vi "Write UUID.vi"(8 "error in (no error)":errorcluster, 10 "UUID":string, 11 "UI View in":refnum<class "UI View.lvclass">) -> (0 "error out":errorcluster, 3 "UI View out":refnum<class "UI View.lvclass">)   [LabVIEW 2013, in "SET Project Editor.lvlib" / "UI View.lvclass"]
uses:
  UI View.lvclass
  UI View.lvclass/UI View.ctl
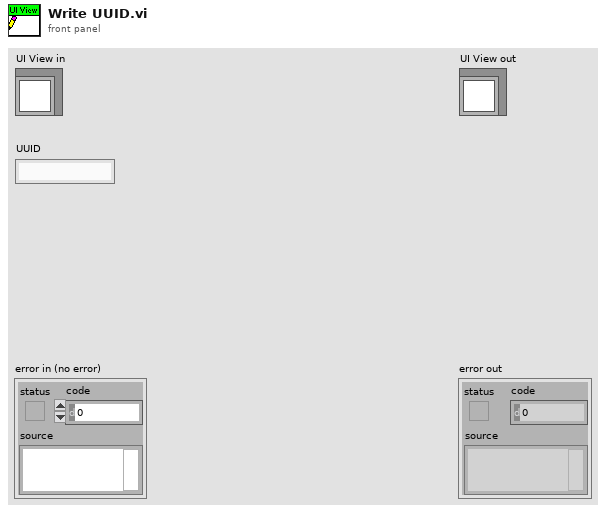
[diagram p1: front panel]
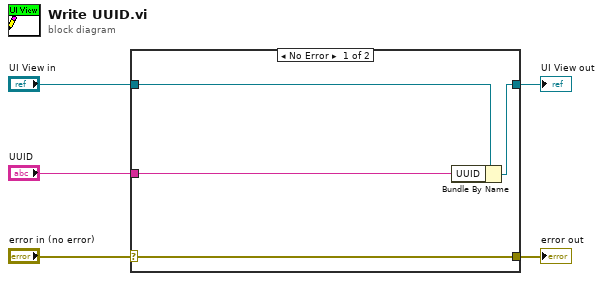
[diagram p0: block diagram]
diagram:
  n1 = case shown="No Error" "error in (no error)" {
    selector: "error in (no error)" -> [w9 w10]
    tunnel: [w9 w10] -> w4
    tunnel: [w7 w11] -> w2
    tunnel: "UI View in" -> [w8 w11]
    tunnel: "UUID" -> [w6 _]
    frame No Error {
      n2 = Bundle By Name(cluster=w8, "UUID"=w6) -> (w7:refnum<class "UI View.lvclass">)
    }
    frame Error {
    }
  }
  "error out" <- w4
  "UI View out" <- w2
